vi "DateAndTime.vi"() -> ()   [LabVIEW 2020]
doc: "This VI have examples of LabVIEW Timestamp, date and time. Comments in polish language."
uses:
  <vilib>/Utility/miscctls.llb/LVDateTimeRec.ctl
panel:
  out "Date time rec":T1 caption="Konwersja przez \"Seconds to Date/Time\""
  out "Resulting string":string="0" caption="Konwersja przez \"Format into string\""
  in  "Switch":bool
  in  "Time Stamp":timestamp=timestamp(1 s since 1904-01-01) format="%^<%.3X\n%x>T"
  out "Absolute time":dbl=-3600.0 caption="Czas absolutny" format="%<%H:%M:%S>T"
  out "Number of seconds":dbl caption="Liczba sekund od 00:00,000 01.01.1904"
  out "Relative time":dbl caption="Czas relatywny" format="%<%H:%M:%S>t"
  out "Date string":string="0"
  out "Time string":string="0"
  out "Date/time string":string="0" caption="Konwersja na string przez \"Fromat Date and Time String"
  # "Timestamp"
  # "Aktualny czas"
  # "Konwersja przez Get Date/Time String"
  # "Konwersja przez \"To DBL\""
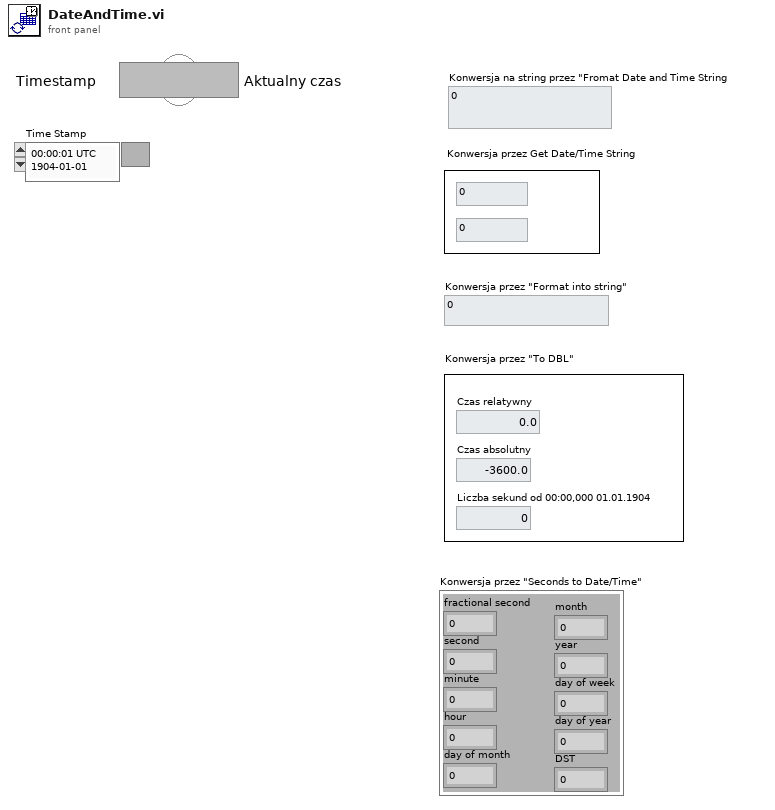
[diagram p1: front panel]
types:
  T1 = typedef "LVDateTimeRec.ctl" = cluster{"fractional second":dbl, "second":i32, "minute":i32, "hour":i32, "day of month":i32, "month":i32, "year":i32, "day of week":i32, "day of year":i32, "DST":i32}
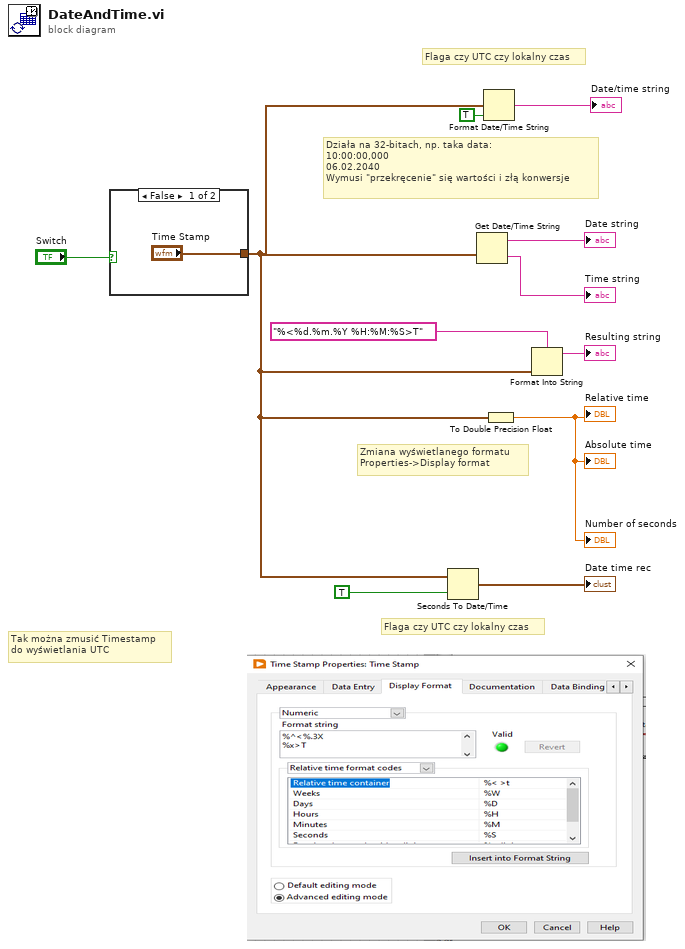
[diagram p0: block diagram]
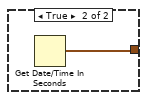
[diagram p2: hidden frame]
diagram:
  # "Tak można zmusić Timestamp\ndo wyświetlania UTC"
  # "Zmiana wyświetlanego formatu\nProperties->Display format"
  # "Flaga czy UTC czy lokalny czas"
  # "Flaga czy UTC czy lokalny czas"
  # "Działa na 32-bitach, np. taka data:\n10:00:00,000\n06.02.2040\nWymusi \"przekręcenie\" się wartości i złą konwersje"
  n1 = case shown="False" "Switch" {
    tunnel: ["Time Stamp" w13] -> w4
    frame False {
    }
    frame True {
      n2 = Get Date/Time In Seconds() -> (seconds since 1Jan1904=w13:timestamp)
    }
  }
  n3 = Seconds To Date/Time(time stamp (now)=w4, to UTC (F)=TRUE) -> (date time rec=→"Date time rec":T1)
  n4 = Get Date/Time String(seconds (now)=w4) -> (date string=→"Date string":string, time string=→"Time string":string)  [unwired: 2 in]
  n5 = Format Date/Time String(seconds (now)=w4, UTC format=TRUE) -> (date/time string=→"Date/time string":string)  [unwired: 1 in]
  n6 = To Double Precision Float(number=w4) -> (double precision float=→"Relative time" →"Number of seconds" →"Absolute time":dbl)
  n7 = Format Into String(format string="%<%d.%m.%Y %H:%M:%S>T", w4) -> (resulting string=→"Resulting string":string)  [unwired: 2 in, 1 out]
